vi "APS get position.vi"(8 "error in (no error)":errorcluster caption="错误输入（无错误）", 11 "Axis_ID":i32) -> (0 "error out":errorcluster caption="错误输出", 1 "Position":i32, 3 "function return":i32)   [LabVIEW 2012, in "APS168.lvlib"]
doc: "I32 FNTYPE APS_get_position( I32 Axis_ID, I32 *Position );"
uses:
  APS168.lvlib
  APS168.dll
panel:
  out "Axis_ID2":i32
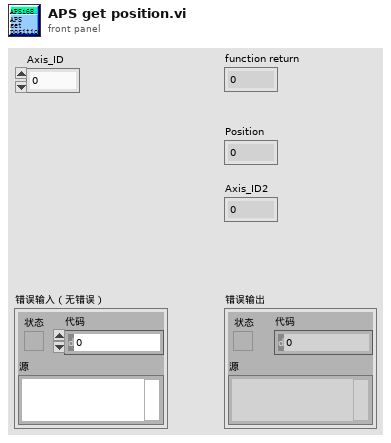
[diagram p1: front panel]
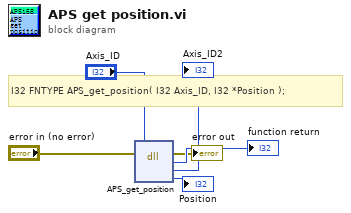
[diagram p0: block diagram]
diagram:
  # "I32 FNTYPE APS_get_position( I32 Axis_ID, I32 *Position );"
  n1 = dll-call lib="PTH1/abs E\t冲压机LLB运动204cAPS168.*" fn="APS_get_position"(error in="error in (no error)", "Axis_ID"="Axis_ID") -> (error out=→"error out":errorcluster, "return type"=→"function return":i32, "Axis_ID"=→"Axis_ID2":i32, "Position"=→"Position":i32)  [unwired: 3 in, 1 out]
